vi "mouse_and_cheese_maze.vi"() -> ()   [LabVIEW 2016]
doc: "Places a mouse in the first open column and cheese in the last column of the maze. Then mouse can trace the cheese by left or right hand method.\n\nMuhannad Alghamdi\nCSUSB Physics 350"
uses:
  typedefs/cell_typedef.ctl
  typedefs/state.ctl
  typedefs/action_start.ctl
panel:
  in  "Restart":bool
  out "Solution Count":dbl
  out "State Count":i32
  in  "Stop":bool
  out "Current State":T1={"State"=enum."sense", "Maze"=[[FALSE, FALSE, FALSE, FALSE, FALSE, FALSE, FALSE, FALSE, FALSE], [FALSE, FALSE, FALSE, FALSE, FALSE, FALSE, FALSE, FALSE, FALSE], [FALSE, FALSE, FALSE, FALSE, FALSE, FALSE, FALSE, FALSE, FALSE], [FALSE, FALSE, FALSE, FALSE, FALSE, FALSE, FALSE, FALSE, FALSE], [TRUE, TRUE, FALSE, FALSE, FALSE, FALSE, FALSE, TRUE, TRUE], [FALSE, FALSE, FALSE, FALSE, FALSE, FALSE, FALSE, FALSE, FALSE], [FALSE, FALSE, FALSE, FALSE, FALSE, FALSE, FALSE, FALSE, FALSE], [FALSE, FALSE, FALSE, FALSE, FALSE, FALSE, FALSE, FALSE, FALSE], [FALSE, FALSE, FALSE, FALSE, FALSE, FALSE, FALSE, FALSE, FALSE]], "Runner Row"=4, "Runner Column"=0, "Runner Direction"=enum."east", "Sense"={"wall in front"=TRUE, "wall to left"=FALSE, "wall to right"=TRUE, "wall behind"=TRUE, "exit column"=FALSE}, "Hand"=enum."Left-handed"}
  out "Maze with R`unner":T3[][](array[typedef])=[[{"open"=FALSE, "runner"=0}, {"open"=FALSE, "runner"=0}, {"open"=FALSE, "runner"=0}, {"open"=FALSE, "runner"=0}, {"open"=FALSE, "runner"=0}, {"open"=FALSE, "runner"=0}, {"open"=FALSE, "runner"=0}, {"open"=FALSE, "runner"=0}, {"open"=FALSE, "runner"=0}], [{"open"=FALSE, "runner"=0}, {"open"=FALSE, "runner"=0}, {"open"=FALSE, "runner"=0}, {"open"=FALSE, "runner"=0}, {"open"=FALSE, "runner"=0}, {"open"=FALSE, "runner"=0}, {"open"=FALSE, "runner"=0}, {"open"=FALSE, "runner"=0}, {"open"=FALSE, "runner"=0}], [{"open"=FALSE, "runner"=0}, {"open"=FALSE, "runner"=0}, {"open"=FALSE, "runner"=0}, {"open"=FALSE, "runner"=0}, {"open"=FALSE, "runner"=0}, {"open"=FALSE, "runner"=0}, {"open"=FALSE, "runner"=0}, {"open"=FALSE, "runner"=0}, {"open"=FALSE, "runner"=0}], [{"open"=FALSE, "runner"=0}, {"open"=FALSE, "runner"=0}, {"open"=FALSE, "runner"=0}, {"open"=FALSE, "runner"=0}, {"open"=FALSE, "runner"=0}, {"open"=FALSE, "runner"=0}, {"open"=FALSE, "runner"=0}, {"open"=FALSE, "runner"=0}, {"open"=FALSE, "runner"=0}], [{"open"=TRUE, "runner"=1}, {"open"=TRUE, "runner"=0}, {"open"=FALSE, "runner"=0}, {"open"=FALSE, "runner"=0}, {"open"=FALSE, "runner"=0}, {"open"=FALSE, "runner"=0}, {"open"=FALSE, "runner"=0}, {"open"=TRUE, "runner"=0}, {"open"=TRUE, "runner"=0}], [{"open"=FALSE, "runner"=0}, {"open"=FALSE, "runner"=0}, {"open"=FALSE, "runner"=0}, {"open"=FALSE, "runner"=0}, {"open"=FALSE, "runner"=0}, {"open"=FALSE, "runner"=0}, {"open"=FALSE, "runner"=0}, {"open"=FALSE, "runner"=0}, {"open"=FALSE, "runner"=0}], [{"open"=FALSE, "runner"=0}, {"open"=FALSE, "runner"=0}, {"open"=FALSE, "runner"=0}, {"open"=FALSE, "runner"=0}, {"open"=FALSE, "runner"=0}, {"open"=FALSE, "runner"=0}, {"open"=FALSE, "runner"=0}, {"open"=FALSE, "runner"=0}, {"open"=FALSE, "runner"=0}], [{"open"=FALSE, "runner"=0}, {"open"=FALSE, "runner"=0}, {"open"=FALSE, "runner"=0}, {"open"=FALSE, "runner"=0}, {"open"=FALSE, "runner"=0}, {"open"=FALSE, "runner"=0}, {"open"=FALSE, "runner"=0}, {"open"=FALSE, "runner"=0}, {"open"=FALSE, "runner"=0}], [{"open"=FALSE, "runner"=0}, {"open"=FALSE, "runner"=0}, {"open"=FALSE, "runner"=0}, {"open"=FALSE, "runner"=0}, {"open"=FALSE, "runner"=0}, {"open"=FALSE, "runner"=0}, {"open"=FALSE, "runner"=0}, {"open"=FALSE, "runner"=0}, {"open"=FALSE, "runner"=0}]]
  in  "Hand":enum32{"Left-handed", "Right-handed"}(radio)
  in  "Milliseconds to Wait":u32(slide)=50 scale=1.0..1000.0
  in  "Maze to Run":bool[][](array[boolean])=[[FALSE, FALSE, FALSE, FALSE, FALSE, FALSE, FALSE, FALSE, FALSE], [FALSE, TRUE, TRUE, TRUE, FALSE, FALSE, FALSE, FALSE, FALSE], [FALSE, FALSE, FALSE, TRUE, FALSE, TRUE, TRUE, TRUE, FALSE], [FALSE, TRUE, TRUE, TRUE, FALSE, TRUE, FALSE, TRUE, FALSE], [TRUE, TRUE, FALSE, TRUE, FALSE, TRUE, FALSE, TRUE, TRUE], [FALSE, FALSE, FALSE, TRUE, FALSE, TRUE, FALSE, FALSE, FALSE], [FALSE, FALSE, TRUE, TRUE, TRUE, TRUE, TRUE, FALSE, FALSE], [FALSE, TRUE, TRUE, FALSE, FALSE, FALSE, TRUE, FALSE, FALSE], [FALSE, FALSE, FALSE, FALSE, FALSE, FALSE, FALSE, FALSE, FALSE]]
  # "Mouse and Cheese Maze"
  # "Muhannad Alghamdi\nCSUSB Physics 350\nProject 4"
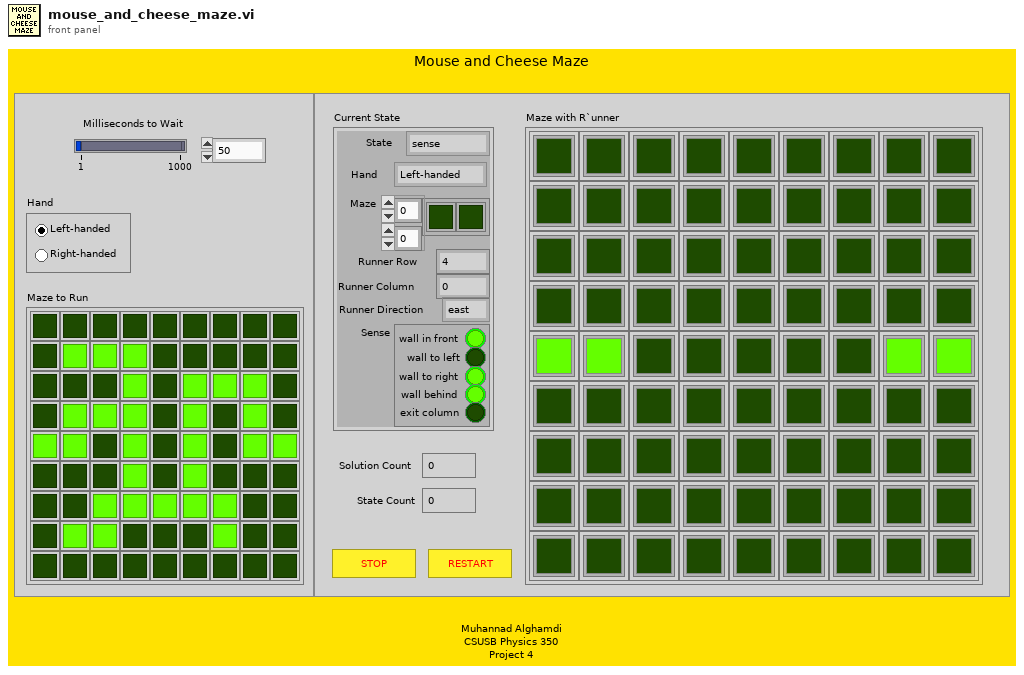
[diagram p1: front panel]
types:
  T1 = typedef "state.ctl" = cluster{"State":T2, "Maze":bool[][], "Runner Row":i32, "Runner Column":i32, "Runner Direction":enum16{"east", "north", "west", "south"}, "Sense":cluster{"wall in front":bool, "wall to left":bool, "wall to right":bool, "wall behind":bool, "exit column":bool}, "Hand":enum16{"Left-handed", "Right-handed"}}
  T2 = typedef "action_start.ctl" = enum16{"sense", "decide", "step", "pivot right", "pivot left", "stop"}
  T3 = typedef "cell_typedef.ctl" = cluster{"open":bool, "runner":u16}
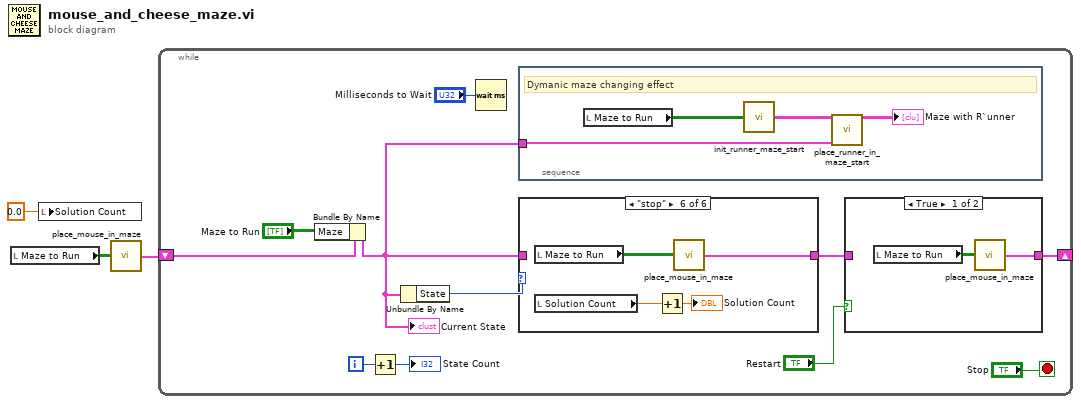
[diagram p0: block diagram]
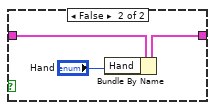
[diagram p2: hidden frame]
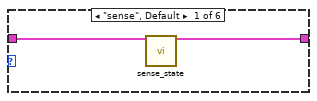
[diagram p3: hidden frame]
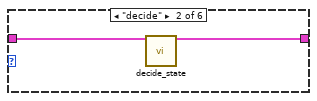
[diagram p4: hidden frame]
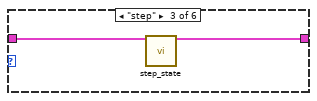
[diagram p5: hidden frame]
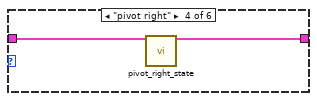
[diagram p6: hidden frame]
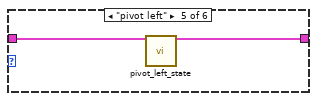
[diagram p7: hidden frame]
diagram:
  n1 = local read "Maze to Run"() -> (w1:bool[][])
  n2 = local write "Solution Count"(0.0 ("Numeric")) -> ()
  n3 = call "place_mouse_in_maze.vi"("Maze to Run"=w1) -> ("output cluster"=w3:T1)
  n4 = while {
    shift-right: [w8] -> _
    shift-left: w3 -> [w6]
    i -> [w12]
    stop <- "Stop" stop-if-true
    n5 = Bundle By Name(cluster=w6, "Maze"="Maze to Run") -> (w5:T1)
    "Current State" <- w5
    n6 = Increment(x=w12) -> (x+1=→"State Count":i32)
    n7 = Unbundle By Name(w5) -> ("State"=w14:T2)
    n8 = Wait (ms)(milliseconds to wait="Milliseconds to Wait") -> ()  [unwired: 1 out]
    n9 = stacked-sequence {
      tunnel: w5 -> [w22]
      frame #0 {
        # "Dymanic maze changing effect"
        n10 = local read "Maze to Run"() -> (w21:bool[][])
        n11 = call "init_runner_maze_start.vi"("maze array"=w21) -> ("maze with runner array"=w20:T3[][])  [unwired: 14 in]
        n12 = call "place_runner_in_maze_start.vi"("maze with runner in"=w20, "state"=w22) -> ("maze with runner out"=→"Maze with R`unner":T3[][])  [unwired: 13 in]
      }
    }
    n13 = case shown="\"stop\"" w14 {
      tunnel: [w25 w27 w29 w31 w33 w37] -> w9
      tunnel: w5 -> [w24 w26 w28 w30 w32 _]
      frame "sense", Default {
        n14 = call "sense_state.vi"("state in"=w24) -> ("state out"=w25:T1)  [unwired: 14 in]
      }
      frame "decide" {
        n15 = call "decide_state.vi"("state in"=w26) -> ("state out"=w27:T1)  [unwired: 14 in]
      }
      frame "step" {
        n16 = call "step_state.vi"("state in"=w28) -> ("state out"=w29:T1)  [unwired: 14 in]
      }
      frame "pivot right" {
        n17 = call "pivot_right_state.vi"("state in"=w30) -> ("state out"=w31:T1)  [unwired: 14 in]
      }
      frame "pivot left" {
        n18 = call "pivot_left_state.vi"("state in"=w32) -> ("state out"=w33:T1)  [unwired: 14 in]
      }
      frame "stop" {
        n19 = local read "Maze to Run"() -> (w36:bool[][])
        n20 = local read "Solution Count"() -> (w34:dbl)
        n21 = Increment(x=w34) -> (x+1=→"Solution Count":dbl)
        n22 = call "place_mouse_in_maze.vi"("Maze to Run"=w36) -> ("output cluster"=w37:T1)
      }
    }
    n23 = case shown="True" "Restart" {
      tunnel: w9 -> [_ w19]
      tunnel: [w15 w18] -> w8
      frame True {
        n24 = local read "Maze to Run"() -> (w16:bool[][])
        n25 = call "place_mouse_in_maze.vi"("Maze to Run"=w16) -> ("output cluster"=w15:T1)
      }
      frame False {
        n26 = Bundle By Name(cluster=w19, "Hand"="Hand") -> (w18:T1)
      }
    }
  }
